vi "Send Get Table Object.vi"(6 "timeout in ms (-1)":i32=-1, 7 "Message Priority (Normal)":T2=enum."Normal", 8 "error in (no error)":errorcluster, 10 "Form ID":T1, 11 "Message Enqueuer":refnum<class "Message Enqueuer.lvclass">) -> (0 "error out":errorcluster, 2 "Table":refnum<class "Basic Table.lvclass">, 3 "Message Enqueuer out":refnum<class "Message Enqueuer.lvclass">, 4 "timed out?":bool)   [LabVIEW 2020, in "Form Server Interfaces.lvlib" / "Get Table Object Msg.lvclass"]
doc: "This VI sends the message to an actor."
uses:
  Get Table Object Msg.lvclass
  <vilib>/ActorFramework/Message Enqueuer/Message Enqueuer.lvclass
  <vilib>/ActorFramework/Message Enqueuer/Message Priority.ctl
  Autoclose manager/Form ID.ctl
  Database OOP/Table Libraries/Basic Table/Basic Table Class/Basic Table.lvclass
  C:/Program Files (x86)/National Instruments/LabVIEW 2020/vi.lib/ActorFramework/Reply Msg/Reply Msg.lvclass
  Get Table Object Msg.lvclass/Get Table Object Msg.ctl
  <vilib>/ActorFramework/Reply Msg/Reply Msg.lvclass/Reply Msg.ctl
  <vilib>/ActorFramework/Message Enqueuer/Message Enqueuer.lvclass/Message Enqueuer.ctl
  <vilib>/ActorFramework/Message Enqueuer/Enqueue.vi
  <vilib>/ActorFramework/Reply Msg/Reply Msg.lvclass
  C:/Program Files (x86)/National Instruments/LabVIEW 2020/vi.lib/ActorFramework/Message/Message.lvclass
  <vilib>/ActorFramework/Message Priority Queue/Priority Enqueue.vi
  Form Server Interfaces.lvlib
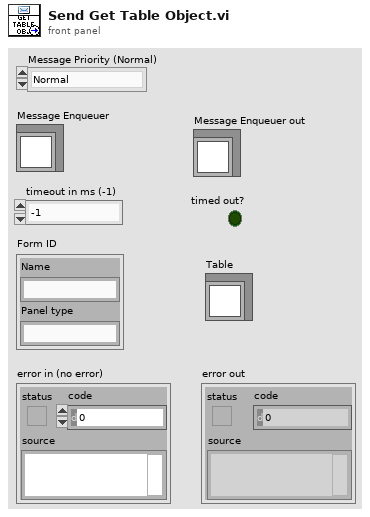
[diagram p1: front panel]
types:
  T1 = typedef "Form Server Interfaces.lvlib/Form ID.ctl" = cluster{"Name":string, "Panel type":string}
  T2 = typedef "Panel Form Controller.lvlib/Actor Framework.lvlib/Message Enqueuer.lvclass/Message Priority.ctl" = enum16{"Low", "Normal", "High"}
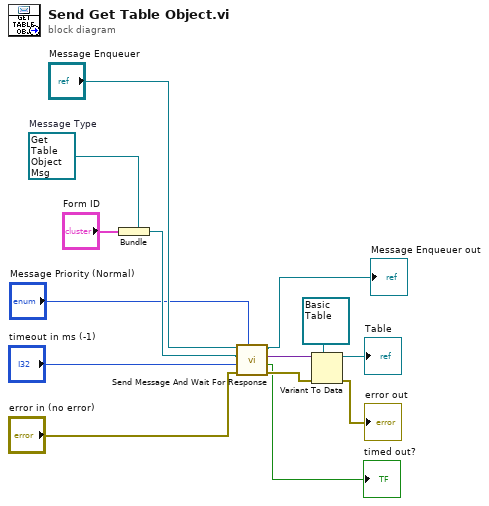
[diagram p0: block diagram]
diagram:
  w14 = refnum<class "Get Table Object Msg.lvclass"> refnum  # Message Type
  n1 = Bundle(cluster=w14, "Form ID") -> (w11:refnum<class "Get Table Object Msg.lvclass">)
  n2 = call <vilib>:"Send Message And Wait For Response.vi"("Message Priority (Normal)"="Message Priority (Normal)", "error in (no error)"="error in (no error)", "timeout in ms (-1)"="timeout in ms (-1)", "Original Message"=w11, "Message Enqueuer in"="Message Enqueuer") -> ("error out"=w6:errorcluster, "timed out?"=→"timed out?":bool, "Reply"=w5:variant, "Message Enqueuer out"=→"Message Enqueuer out":refnum<class "Message Enqueuer.lvclass">)  [unwired: 3 in]
  n3 = Variant To Data(error in=w6, type=refnum<class "Basic Table.lvclass"> refnum ("Table"), Variant=w5) -> (data=→"Table":refnum<class "Basic Table.lvclass">, error out=→"error out":errorcluster)
